vi "DelayLineWait.vi"(0 "Inst_param":T1) -> ()   [LabVIEW 2013]
uses:
  Drivers/Get Parameter.ctl
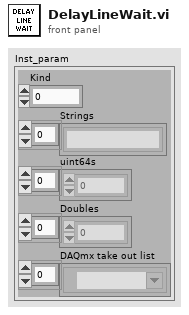
[diagram p1: front panel]
types:
  T1 = cluster{"Kind":u16, "Strings":string[], "uint64s":u64[], "Doubles":dbl[], "DAQmx take out list":refnum<k21>[]}
  T2 = typedef "Get Parameter.ctl" = enum16{"Acceleration (A)", "Baud Rate (BD)", "Busy Flag (BY)", "Counter 1 (C1)", "Counter 2 (C2)", "Check Sum Enable (CK)", "Clock Mode (CM)", "Clock Mode Ratio (CR)", "Clock Mode Out Step Width (CW)", "Deceleration (D)", "Digital Filtering, Input 1 (D1)", "Digital Filtering, Input 2 (D2)", "Digital Filtering, Input 3 (D3)", "Digital Filtering, Input 4 (D4)", "Digital Filtering, Input 5 (D5)", "Digital Filtering, Input 9 (D9)", "Digital Filtering, Input 10 (D10)", "Digital Filtering, Input 11 (D11)", "Digital Filtering, Input 12 (D12)", "Deadband (DB)", "Enable/Disable Drive (DE)", "Device Name (DN)", "End Program Execution (E)", "Encoder Function Enable (EE)", "Encoder Lines (EL)", "Error Flag (EF)", "Error Variable (ER)", "Echo Mode (EM)", "Escape (ES)", "Execute Program at Address (EX)", "Hold Current (HC)", "Hold Current Delay Time (HI)", "Input 1 (I1)", "Input 2 (I2)", "Input 3 (I3)", "Input 4 (I4)", "Input 5 Analog (I5)", "Input 6 Encoder Index (I6)", "Input 9 (I9)", "Input 10 (I10)", "Input 11 (I11)", "Input 12 (I12)", "Input Low Byte (1-4) (IL)", "Input High Byte (9-12) (IH)", "Inputs Total (1-4,9-12) (IN)", "Internal Temperature (IT)", "Jog Enable (JE)", "Limit Stop Mode (LM)", "MicroStepping Select (MS)", "Motor Settling Delay Time (MT)", "Moving Flag (MV)", "Output 1 (O1)", "Output 2 (O2)", "Output 3 (O3)", "Output 4 (O4)", "Output 9 (O9)", "Output 10 (O10)", "Output 11 (O11)", "Output 12 (O12)", "Output High Byte (9-12) (OH)", "Output Low Byte (1-4) (OL)", "Output Total (1-4 and 9-12) (OT)", "Position Captured at Trip (PC)", "Position Maintenance (PM)", "Part Number (PN)", "Party Mode (PY)", "Register 1 (R1)", "Register 2 (R2)", "Register 3 (R3)", "Register 4 (R4)", "Run Current (RC)", "Serial Number (SN)", "Stall Flag (ST)", "Stall Factor (SF)", "Stall Mode Set (SM)", "User Variables (UV)", "Velocity (V)", "Velocity Changing Flag (VC)", "Velocity Initial (VI)", "Version, Firmware (VR)", "Velocity Maximum (VM)"}
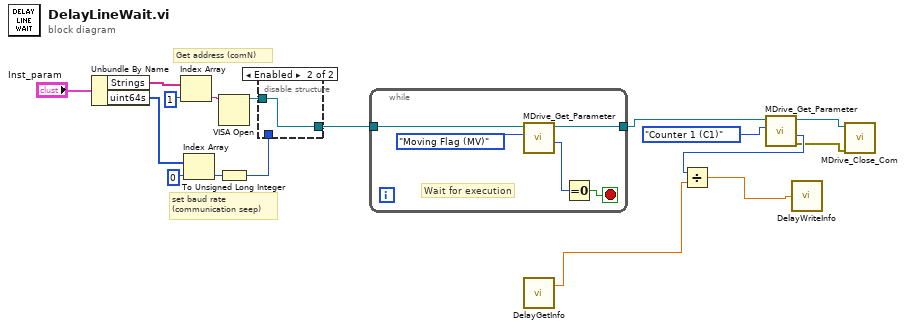
[diagram p0: block diagram]
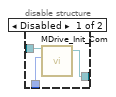
[diagram p2: hidden frame]
diagram:
  # "Get address (comN)"
  # "set baud rate\n(communication seep)"
  n1 = Unbundle By Name("Inst_param") -> ("Strings"=w17:string[], "uint64s"=w10:u64[])
  n2 = Index Array(array=w17, index=1) -> (element=w15:string)
  n3 = Index Array(array=w10, index=0) -> (element=w12:u64)
  n4 = VISA Open(VISA resource name=w15) -> (VISA resource name=w14:refnum<visa-resource-name>)  [unwired: 4 in, 1 out]
  n5 = To Unsigned Long Integer(number=w12) -> (unsigned 32bit integer=w11:u32)
  n6 = disable-structure shown="Enabled" {
    disable-tunnel: w14 -> [w20 w21]
    disable-tunnel: w11 -> [w19 _]
    disable-tunnel: [w18 w21] -> w8
    frame Disabled {
      n7 = call "MDrive_Init_Com.vi"("VISA resource name"=w20, "baud rate"=w19) -> ("VISA resource name out"=w18:refnum<visa-resource-name>)  [unwired: 5 in, 1 out]
    }
    frame Enabled {
    }
  }
  n8 = while {
    tunnel: w8 -> [w23]
    tunnel: [w22] -> w5
    stop <- w24 stop-if-true
    # "Wait for execution"
    n9 = call "MDrive_Get_Parameter.vi"("Get Parameter"=Get_Parameter."Moving Flag (MV)", "VISA resource name in"=w23) -> ("Parameter Data Numeric"=w25:i32, "VISA resource name out"=w22:refnum<visa-resource-name>)  [unwired: 2 in, 2 out]
    n10 = Equal To 0?(x=w25) -> (x = 0?=w24:bool)
  }
  n11 = call "DelayGetInfo.vi"() -> ("Conversion"=w2:dbl)  [unwired: 2 in, 1 out]
  n12 = call "MDrive_Get_Parameter.vi"("Get Parameter"=Get_Parameter."Counter 1 (C1)", "VISA resource name in"=w5) -> ("error out"=w3:errorcluster, "Parameter Data Numeric"=w6:i32, "VISA resource name out"=w4:refnum<visa-resource-name>)  [unwired: 2 in, 1 out]
  n13 = Divide(x=w6, y=w2) -> (x/y=w1:dbl)
  n14 = call "DelayWriteInfo.vi"("Delay position input (ps)"=w1) -> ()
  n15 = call "MDrive_Close_Com.vi"("error out"=w3, "VISA resource name out"=w4) -> ()  [unwired: 2 in]
